vi "Set Polling Message.vi"(8 "error in (no error)":errorcluster, 10 "Timeout Message":refnum<class "~Message.lvclass">, 11 "Zero Timeout Message Handler in":refnum<class "Zero Timeout Message Handler.lvclass">) -> (0 "error out":errorcluster, 3 "Zero Timeout Message Handler out":refnum<class "Zero Timeout Message Handler.lvclass">)   [LabVIEW 2024, in "Zero Timeout Message Handler.lvlib" / "Zero Timeout Message Handler.lvclass"]
uses:
  Zero Timeout Message Handler.lvclass
  ~Message/~Message.lvclass
  Zero Timeout Message Handler.lvclass/Zero Timeout Message Handler.ctl
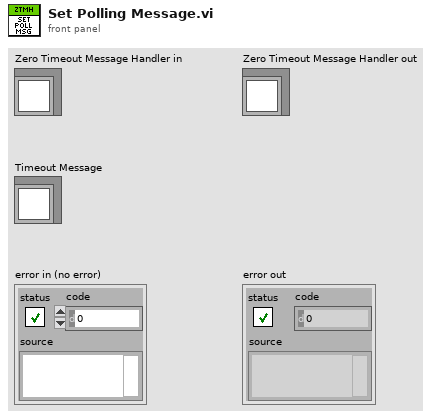
[diagram p1: front panel]
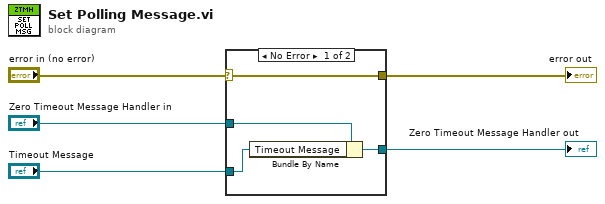
[diagram p0: block diagram]
diagram:
  n1 = case shown="No Error" "error in (no error)" {
    selector: "error in (no error)" -> [w9 w11]
    tunnel: [w9 w11] -> w4
    tunnel: [w6 w10] -> w2
    tunnel: "Zero Timeout Message Handler in" -> [w8 w10]
    tunnel: "Timeout Message" -> [w7 _]
    frame No Error {
      n2 = Bundle By Name(cluster=w8, "Timeout Message"=w7) -> (w6:refnum<class "Zero Timeout Message Handler.lvclass">)
    }
    frame Error {
    }
  }
  "error out" <- w4
  "Zero Timeout Message Handler out" <- w2
